vi "Update FOV FGV.vi"(8 "error in (no error)":errorcluster, 11 "FOV control ref":refnum<vi>) -> (0 "error out":errorcluster)   [LabVIEW 2020]
uses:
  <vilib>/Utility/miscctls.llb/LVStringsAndValuesArrayTypeDef_SGL.ctl
panel:
  out "Strings And Values []":T1
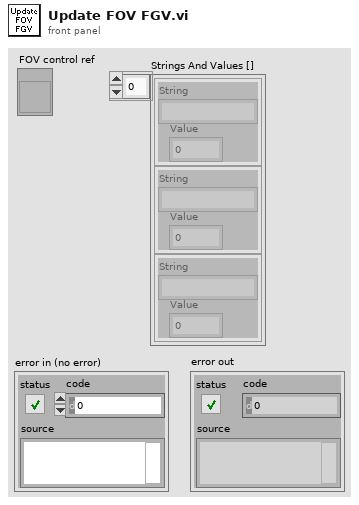
[diagram p1: front panel]
types:
  T1 = typedef "LVStringsAndValuesArrayTypeDef_SGL.ctl" = cluster{"String":string, "Value":sgl}[]
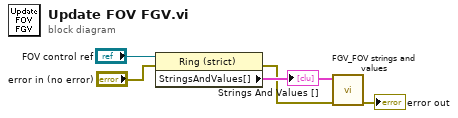
[diagram p0: block diagram]
diagram:
  n1 = property on="Property Node" class="Ring (strict)"(reference="FOV control ref", error in="error in (no error)") -> (error out=w2:errorcluster, "StringsAndValues[]"=w5:T1)  [unwired: 1 out]
  "Strings And Values []" <- w5
  n2 = call "FGV_FOV strings and values.vi"("error in (no error)"=w2, "FOV control Strings And Values"=w5) -> ("error out"=→"error out":errorcluster)  [unwired: 8 in, 1 out]
